vi "iXonMultiTrack.vi"() -> ()   [LabVIEW 2009]
uses:
  <userlib>/atmcd32d.llb/Shutter_type typedef.ctl
panel:
  in  "type":T1
  in  "Time to open or\nclose shutter (ms):":i16=50
  in  "Number of Tracks:":i16=5
  out "Return from TrackGap":i16
  out "Return from BottomTrack":i16
  in  "Track Height:":i16=10
  in  "Track Offset:":i16
  out "Return from SetMultitrack":u16
  in  "Shut Down":bool
  in  "Start Acquisition":bool
  out "Graphical Results":i32[](graph)
  out "Return  from Get Acquired Data":u32
  out "Detector X Pixels":i32
  out "Return from GetStatus":u32
  out "Return from Start Acquisition":u32
  out "Return from CheckTimings Exposure":u32
  out "Calculated Exposure Value":sgl format="%.2f"
  in  "Exposure Time (secs)":sgl=0.05 format="%.2f"
  out "Return from Initialize":u32
  in  "Trigger":u32(ring) items=["Internal", "External"]
  # "Status"
  # "Acquisition Mode: Kinetics\nReadout Mode: MultiTrack Image\nOnly showing one track of data."
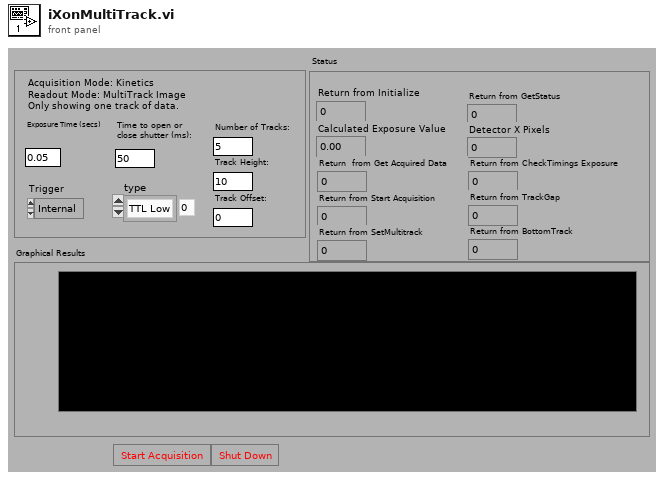
[diagram p1: front panel]
types:
  T1 = typedef "Shutter_type typedef.ctl" = enum16{"TTL Low", "TTL High"}
  T2 = typedef "Error Code Enum typedef.ctl" = enum32{"N/A (0)", "DRV_ERROR_CODES", "DRV_SUCCESS", "DRV_VXDNOTINSTALLED", "DRV_ERROR_SCAN", "DRV_ERROR_CHECK_SUM", "DRV_ERROR_FILELOAD", "DRV_UNKNOWN_FUNC", "DRV_ERROR_VXD_INIT", "DRV_ERROR_ADDRESS", "DRV_ERROR_PAGELOCK", "DRV_ERROR_PAGEUNLOCK", "DRV_ERROR_BOARDTEST", "DRV_ERROR_ACK", "DRV_ERROR_UP_FIFO", "DRV_ERROR_PATTERN", "N/A (16)", "DRV_ACQUISITION_ERRORS", "DRV_ACQ_BUFFER", "DRV_ACQ_DOWNFIFO_FULL", "DRV_PROC_UNKONWN_INSTRUCTION", "DRV_ILLEGAL_OP_CODE", "DRV_KINETIC_TIME_NOT_MET", "DRV_ACCUM_TIME_NOT_MET", "DRV_NO_NEW_DATA", "N/A (25)", "DRV_SPOOLERROR", "N/A (27)", "N/A (28)", "N/A (29)", "N/A (30)", "N/A (31)", "N/A (32)", "DRV_TEMPERATURE_CODES", "DRV_TEMPERATURE_OFF", "DRV_TEMPERATURE_NOT_STABILIZED", "DRV_TEMPERATURE_STABILIZED", "DRV_TEMPERATURE_NOT_REACHED", "DRV_TEMPERATURE_OUT_RANGE", "DRV_TEMPERATURE_NOT_SUPPORTED", "DRV_TEMPERATURE_DRIFT", "N/A (41)", "N/A (42)", "N/A (43)", "N/A (44)", "N/A (45)", "N/A (46)", "N/A (47)", "N/A (48)", "DRV_GENERAL_ERRORS", "DRV_INVALID_AUX", "DRV_COF_NOTLOADED", "DRV_FPGAPROG", "DRV_FLEXERROR", "DRV_GPIBERROR", "N/A (55)", "N/A (56)", "N/A (57)", "N/A (58)", "N/A (59)", "N/A (60)", "N/A (61)", "N/A (62)", "N/A (63)", "DRV_DATATYPE", "DRV_DRIVER_ERRORS", "DRV_P1INVALID", "DRV_P2INVALID", "DRV_P3INVALID", "DRV_P4INVALID", "DRV_INIERROR", "DRV_COFERROR", "DRV_ACQUIRING", "DRV_IDLE", "DRV_TEMPCYCLE", "DRV_NOT_INITIALIZED", "DRV_P5INVALID", "DRV_P6INVALID", "DRV_INVALID_MODE", "DRV_INVALID_FILTER", "DRV_I2CERRORS", "DRV_I2CDEVNOTFOUND", "DRV_I2CTIMEOUT", "DRV_P7INVALID", "N/A (84)", "N/A (85)", "N/A (86)", "N/A (87)", "N/A (88)", "N/A (89)", "DRV_IOCERROR", "DRV_VRMVERSIONERROR"}
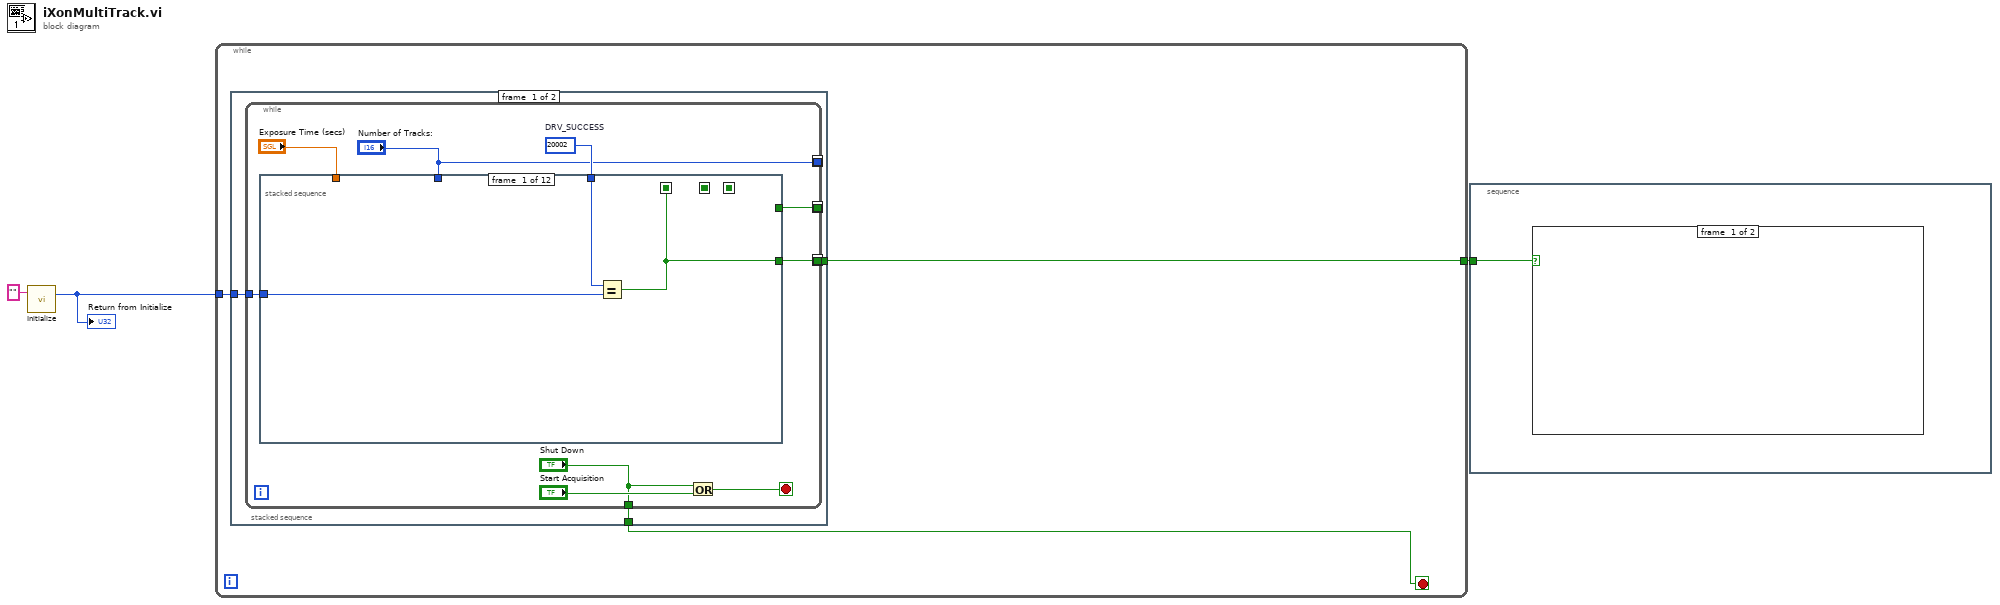
[diagram p0: block diagram]
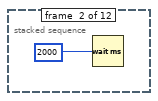
[diagram p2: hidden frame]
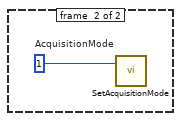
[diagram p4: hidden frame]
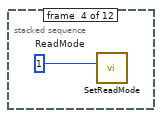
[diagram p5: hidden frame]
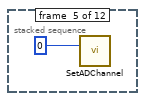
[diagram p6: hidden frame]
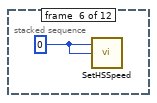
[diagram p7: hidden frame]
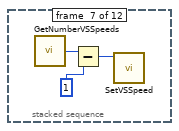
[diagram p8: hidden frame]
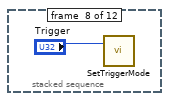
[diagram p9: hidden frame]
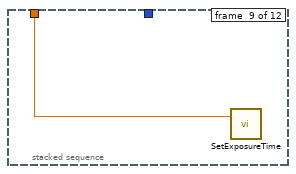
[diagram p10: hidden frame]
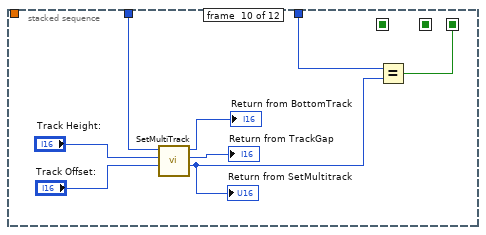
[diagram p11: hidden frame]
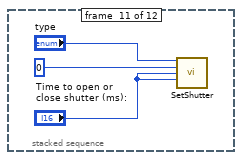
[diagram p12: hidden frame]
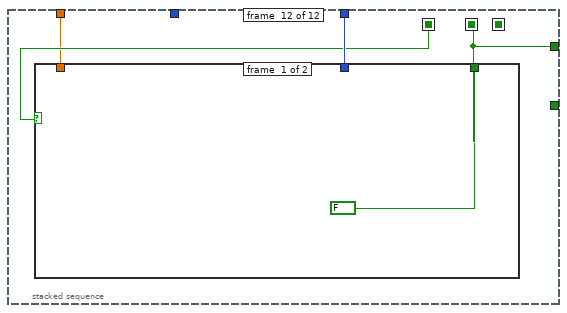
[diagram p13: hidden frame]
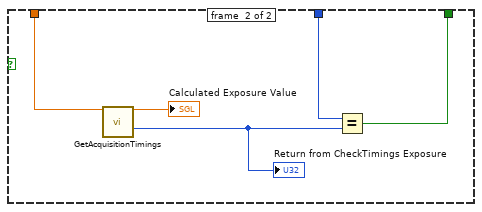
[diagram p14: hidden frame]
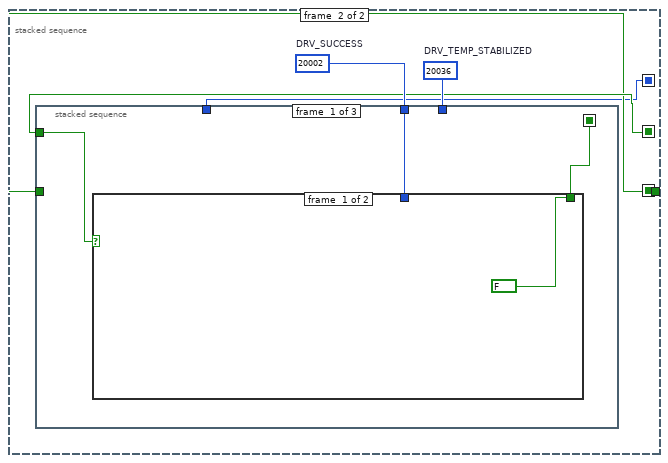
[diagram p15: hidden frame]
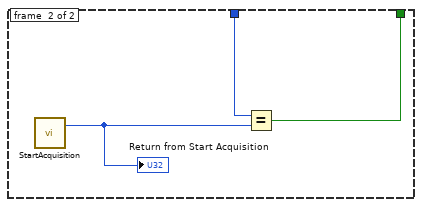
[diagram p16: hidden frame]
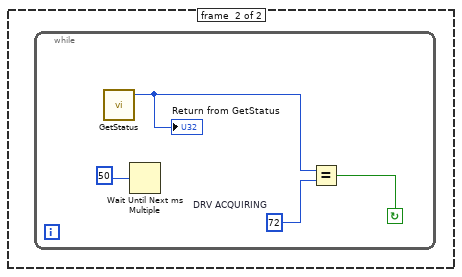
[diagram p18: hidden frame]
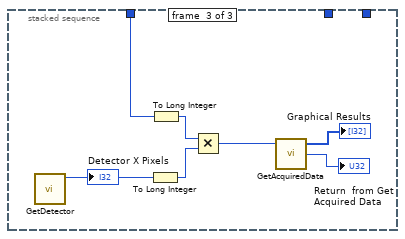
[diagram p19: hidden frame]
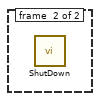
[diagram p20: hidden frame]
diagram:
  n1 = call <userlib>:"Initialize.vi"("directory (\"\")"="" ("directory (\"\")")) -> ("DLL error code"=w2:u32)  [unwired: 1 in, 1 out]
  "Return from Initialize" <- w2
  n2 = while {
    tunnel: w2 -> [w6]
    tunnel: [w5] -> w1
    stop <- w4 stop-if-true
    n3 = stacked-sequence {
      seq-local: [w10 _] -> [_ w58]
      seq-local: [w9 _] -> [_ w57]
      seq-local: [w7 _] -> [_ w56]
      tunnel: w6 -> [w11 _]
      tunnel: [w8 _] -> w4
      tunnel: [_ w57] -> w5
      frame #0 {
        n4 = while {
          tunnel: w11 -> [w18]
          tunnel: [w17] -> w10
          tunnel: [w16] -> w9
          tunnel: ["Shut Down"] -> w8
          tunnel: ["Number of Tracks:"] -> w7
          stop <- w14 stop-if-true
          w19 = 20002  # DRV_SUCCESS
          n5 = stacked-sequence {
            seq-local: [w21 _ _ _ _ _ _ _ _ _ _ _] -> [_ _ w25 _ _ _ _ _ _ _ _ w48]
            seq-local: [_ _ _ _ _ _ _ _ _ _ _ w46] -> [_ _ _ _ _ _ _ _ _ _ _ _]
            seq-local: [_ _ _ _ _ _ _ _ _ w36 _ _] -> [_ _ _ _ _ _ _ _ _ _ _ _]
            tunnel: "Exposure Time (secs)" -> [_ _ _ _ _ _ _ _ w34 _ _ w47]
            tunnel: w19 -> [w23 _ _ _ _ _ _ _ _ w37 _ w49]
            tunnel: w18 -> [w22 _ _ _ _ _ _ _ _ _ _ _]
            tunnel: [_ _ _ _ _ _ _ _ _ _ _ w46] -> w17
            tunnel: [w21 _ _ _ _ _ _ _ _ _ _ _] -> w16
            tunnel: "Number of Tracks:" -> [_ _ _ _ _ _ _ _ _ w35 _ _]
            frame #0 {
              n6 = Equal?(x=w23, y=w22) -> (x = y?=w21:bool)
            }
            frame #1 {
              n7 = Wait (ms)(milliseconds to wait=u32 2000) -> ()  [unwired: 1 out]
            }
            frame #2 {
              n8 = case shown="True" w25 {
                frame #0 {
                }
                frame #1 {
                  w26 = u16 1  # AcquisitionMode
                  n9 = call <userlib>:"SetAcquisitionMode.vi"("mode"=w26) -> ()  [unwired: 1 in, 2 out]
                }
              }
            }
            frame #3 {
              w27 = u16 1  # ReadMode
              n10 = call <userlib>:"SetReadMode.vi"("mode"=w27) -> ()  [unwired: 1 in, 2 out]
            }
            frame #4 {
              n11 = call <userlib>:"SetADChannel.vi"("channel"=0) -> ()  [unwired: 1 in, 2 out]
            }
            frame #5 {
              w29 = 0
              n12 = call <userlib>:"SetHSSpeed.vi"("index"=w29, "type"=w29) -> ()  [unwired: 2 in, 2 out]
            }
            frame #6 {
              n13 = call <userlib>:"GetNumberVSSpeeds.vi"() -> ("DLL error code"=w32:u32)  [unwired: 3 in, 2 out]
              n14 = Subtract(x=w32, y=1) -> (x-y=w30:u32)
              n15 = call <userlib>:"SetVSSpeed.vi"("index"=w30) -> ()  [unwired: 1 in, 2 out]
            }
            frame #7 {
              n16 = call <userlib>:"SetTriggerMode.vi"("mode"="Trigger") -> ()  [unwired: 1 in, 2 out]
            }
            frame #8 {
              n17 = call <userlib>:"SetExposureTime.vi"("time"=w34) -> ()  [unwired: 1 in, 2 out]
            }
            frame #9 {
              n18 = call <userlib>:"SetMultiTrack.vi"("offset"="Track Offset:", "height"="Track Height:", "number"=w35) -> ("DLL error code"=w38:u32, "gap"=→"Return from TrackGap":i32, "bottom"=→"Return from BottomTrack":i32)  [unwired: 1 in, 1 out]
              "Return from SetMultitrack" <- w38
              n19 = Equal?(x=w37, y=w38) -> (x = y?=w36:bool)
            }
            frame #10 {
              n20 = call <userlib>:"SetShutter.vi"("type"="type", "mode"=0, "closingtime"="Time to open or\nclose shutter (ms):", "openingtime"="Time to open or\nclose shutter (ms):") -> ()  [unwired: 10 in, 2 out]
            }
            frame #11 {
              n21 = case shown="True" w48 {
                tunnel: w49 -> [_ w52]
                tunnel: [FALSE w55] -> w46
                tunnel: w47 -> [_ w53]
                frame #0 {
                }
                frame #1 {
                  n22 = call <userlib>:"GetAcquisitionTimings.vi"("exposure input"=w53) -> ("exposure"=→"Calculated Exposure Value":sgl, "DLL error code"=w51:u32)  [unwired: 10 in, 3 out]
                  "Return from CheckTimings Exposure" <- w51
                  n23 = Equal?(x=w52, y=w51) -> (x = y?=w55:bool)
                }
              }
            }
          }
          n24 = Or(x="Shut Down", y="Start Acquisition") -> (x .or. y?=w14:bool)
        }
      }
      frame #1 {
        w59 = 20036  # DRV_TEMP_STABILIZED
        w60 = 20002  # DRV_SUCCESS
        n25 = stacked-sequence {
          seq-local: [w62 _ _] -> [_ w68 _]
          tunnel: w60 -> [w63 _ _]
          tunnel: w59 -> [_ _ _]
          tunnel: w58 -> [w61 _ _]
          tunnel: w57 -> [_ _ _]
          tunnel: w56 -> [_ _ w75]
          frame #0 {
            n26 = case shown="True" w61 {
              tunnel: [FALSE w67] -> w62
              tunnel: w63 -> [_ w66]
              frame #0 {
              }
              frame #1 {
                n27 = call <userlib>:"StartAcquisition.vi"() -> ("DLL error code"=w65:u32)  [unwired: 2 in, 1 out]
                "Return from Start Acquisition" <- w65
                n28 = Equal?(x=w66, y=w65) -> (x = y?=w67:bool)
              }
            }
          }
          frame #1 {
            n29 = case shown="True" w68 {
              frame #0 {
              }
              frame #1 {
                n30 = while {
                  stop <- w71 continue-if-true
                  w70 = u16 72  # DRV ACQUIRING
                  n31 = call <userlib>:"GetStatus.vi"() -> ("status"=w69:T2)  [unwired: 3 in, 2 out]
                  "Return from GetStatus" <- w69
                  n32 = Wait Until Next ms Multiple(millisecond multiple=u32 50) -> ()  [unwired: 1 out]
                  n33 = Equal?(x=w69, y=w70) -> (x = y?=w71:bool)
                }
              }
            }
          }
          frame #2 {
            n34 = call <userlib>:"GetDetector.vi"() -> ("xpixels"=w79:i32)  [unwired: 4 in, 3 out]
            "Detector X Pixels" <- w79
            n35 = To Long Integer(number=w79) -> (32bit integer=w73:i32)
            n36 = To Long Integer(number=w75) -> (32bit integer=w74:i32)
            n37 = Multiply(x=w74, y=w73) -> (x*y=w76:i32)
            n38 = call <userlib>:"GetAcquiredData.vi"("size"=w76) -> ("DLL error code"=→"Return  from Get Acquired Data":u32, "array"=→"Graphical Results":i32[])  [unwired: 2 in, 1 out]
          }
        }
      }
    }
  }
  n39 = stacked-sequence {
    tunnel: w1 -> [w80]
    frame #0 {
      n40 = case shown="True" w80 {
        frame #0 {
        }
        frame #1 {
          n41 = call <userlib>:"ShutDown.vi"() -> ()  [unwired: 2 in, 2 out]
        }
      }
    }
  }
